vi "Filter String Handler_ACAF.vi"(5 "Disable":bool, 6 "Text Colors":cluster{"Text Color":u32, "Text Color 2":u32}={"Text Color"=0, "Text Color 2"=10395294}, 7 "Make key focus?":bool, 8 "error in (no error)":errorcluster, 10 "Default Value":string="Filter...", 11 "String Ref":refnum<vi>) -> (0 "error out":errorcluster)   [LabVIEW 2023]
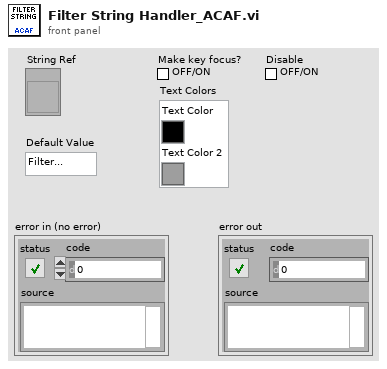
[diagram p1: front panel]
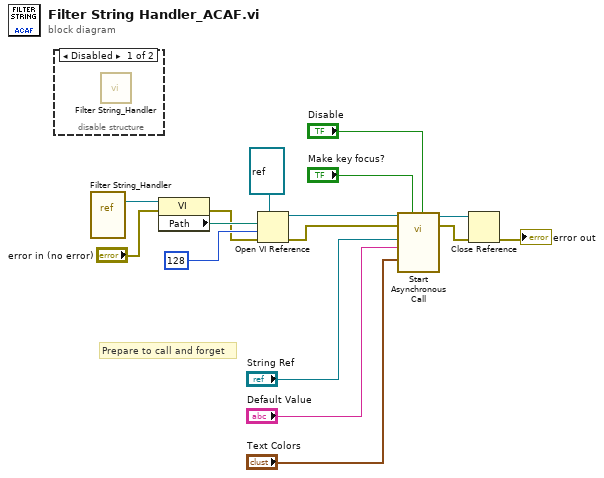
[diagram p0: block diagram]
diagram:
  # "Prepare to call and forget"
  n1 = disable-structure shown="Disabled" {
    frame Disabled {
      n2 = call "Filter String_Handler.vi"() -> ()  [unwired: 12 in]
    }
    frame Enabled {
    }
  }
  n3 = vi-ref "Filter String_Handler.vi"() -> (w16:refnum<vi>)
  n4 = property class="VI"(reference=w16, error in="error in (no error)") -> (error out=w5:errorcluster, "Path"=w12:path)  [unwired: 1 out]
  n5 = Open VI Reference(type specifier VI Refnum (for type only)=refnum<vi> refnum, vi path=w12, options=128, error in (no error)=w5) -> (vi reference=w7:refnum<vi>, error out=w11:errorcluster)  [unwired: 2 in]
  n6 = call-by-ref "Start Asynchronous Call"(reference=w7, error in=w11, "Disable"="Disable", "Text Colors"="Text Colors", "Make key focus?"="Make key focus?", "Default Value"="Default Value", "String Ref"="String Ref") -> (reference out=w10:refnum<vi>, error out=w9:errorcluster)  [unwired: 7 in]
  n7 = Close Reference(reference=w10, error in (no error)=w9) -> (error out=→"error out":errorcluster)
